vi "CreateStandardEvents.vi"(8 "error in":errorcluster) -> (0 "error out":errorcluster, 3 "standard events":T1)   [LabVIEW 2013, in "NISE_CEF_Node.lvclass"]
uses:
  NISE_CEF_Node.lvclass
  StandardEvents.ctl
  UserEventRef.ctl
  Controls/EventCluster.ctl
  NodeChangeEvent.ctl
  NodeRef.ctl
  CacheState.ctl
  RefreshUIEvent.ctl
  StopEvent.ctl
  NISE_CEF_TreeControl.lvlib
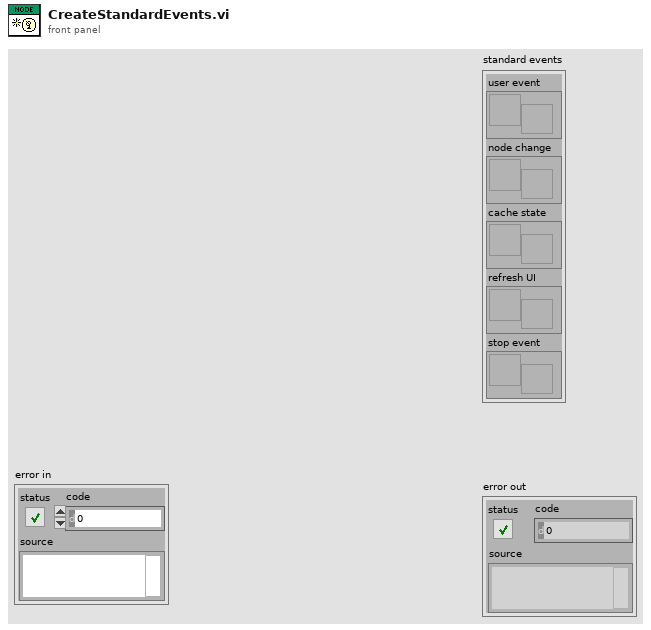
[diagram p1: front panel]
types:
  T1 = typedef "NISE_CEF_Node.lvclass/StandardEvents.ctl" = cluster{"user event":T2, "node change":T3, "cache state":T4, "refresh UI":T5, "stop event":T6}
  T2 = typedef "NISE_CEF_Node.lvclass/UserEventRef.ctl" = refnum<user-event>
  T3 = typedef "NISE_CEF_Node.lvclass/NodeChangeEvent.ctl" = refnum<user-event>
  T4 = typedef "NISE_CEF_Node.lvclass/CacheState.ctl" = refnum<user-event>
  T5 = typedef "NISE_CEF_Node.lvclass/RefreshUIEvent.ctl" = refnum<user-event>
  T6 = typedef "NISE_CEF_Node.lvclass/StopEvent.ctl" = refnum<user-event>
  T7 = typedef "NISE_CEF_Node.lvclass/NodeRef.ctl" = refnum<data-value>
  T8 = typedef "NISE_CEF_TreeControl.lvlib/EventCluster.ctl" = cluster{"command":string, "data":string}
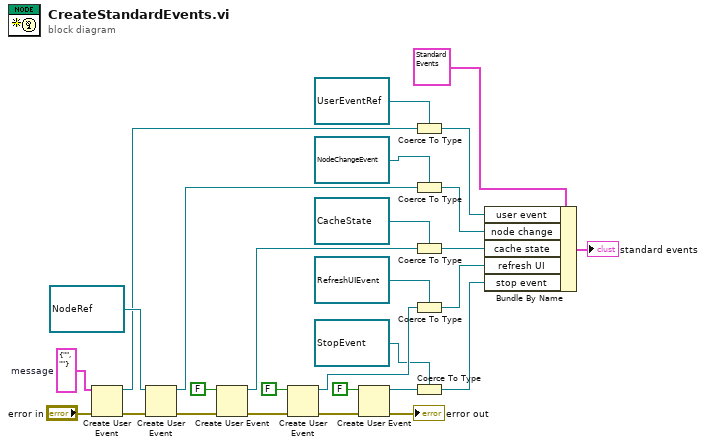
[diagram p0: block diagram]
diagram:
  w20 = T8 {"command"="", "data"=""}  # message
  n1 = Create User Event(user event datatype=w20, error in="error in") -> (user event=w15:refnum<user-event>, error out=w24:errorcluster)
  n2 = Create User Event(user event datatype=T7 refnum ("node ref"), error in=w24) -> (user event=w11:refnum<user-event>, error out=w23:errorcluster)
  n3 = Create User Event(user event datatype=FALSE ("cache state"), error in=w23) -> (user event=w12:refnum<user-event>, error out=w22:errorcluster)
  n4 = Create User Event(user event datatype=FALSE ("refresh UI"), error in=w22) -> (user event=w13:refnum<user-event>, error out=w21:errorcluster)
  n5 = Create User Event(user event datatype=FALSE ("stop"), error in=w21) -> (user event=w14:refnum<user-event>, error out=→"error out":errorcluster)
  n6 = Coerce To Type(0:w15, 1:T2 refnum ("user event")) -> (2:w10:T2)
  n7 = Coerce To Type(0:w11, 1:T3 refnum ("node change")) -> (2:w9:T3)
  n8 = Coerce To Type(0:w12, 1:T4 refnum ("cache state")) -> (2:w8:T4)
  n9 = Coerce To Type(0:w13, 1:T5 refnum ("refresh UI")) -> (2:w7:T5)
  n10 = Coerce To Type(0:w14, 1:T6 refnum ("stop event")) -> (2:w6:T6)
  n11 = Bundle By Name(cluster=T1 {"user event"=refnum, "node change"=refnum, "cache state"=refnum, "refresh UI"=refnum, "stop event"=refnum} ("standard events"), "user event"=w10, "node change"=w9, "cache state"=w8, "refresh UI"=w7, "stop event"=w6) -> (→"standard events":T1)
